vi "myRIO_BRig_Host_formatData_getHeaders_dataTrial.vi"() -> (3 "output_stringArray_dataTrial":string[](array[string]))   [LabVIEW 2014]
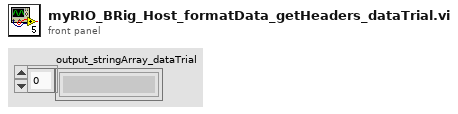
[diagram p1: front panel]
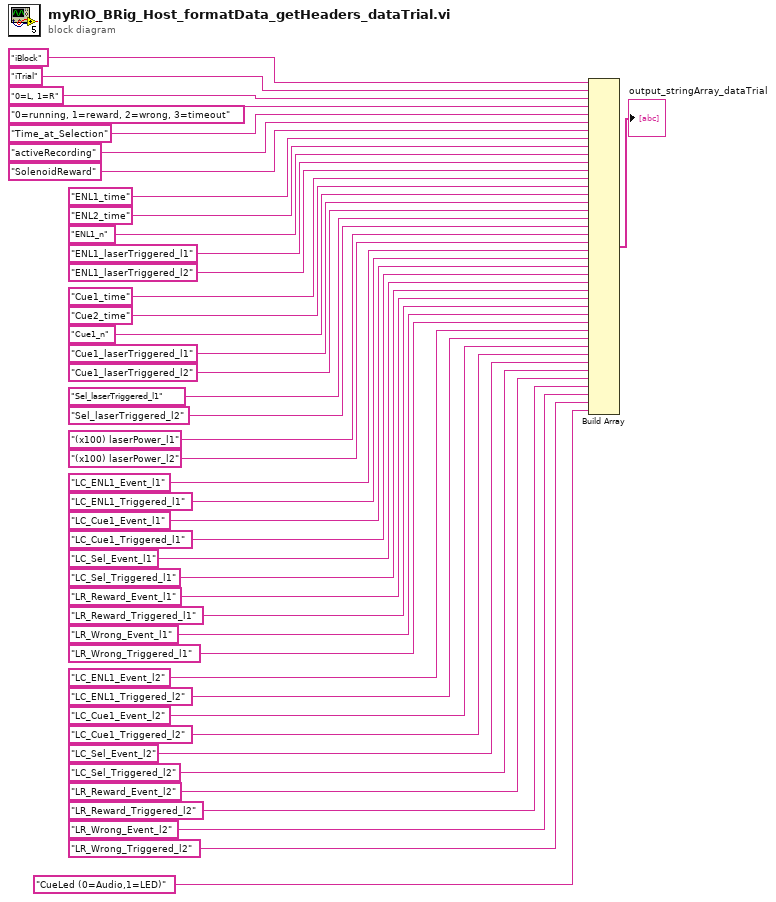
[diagram p0: block diagram]
diagram:
  n1 = Build Array("iBlock", "iTrial", "0=L, 1=R", "0=running, 1=reward, 2=wrong, 3=timeout", "Time_at_Selection", "activeRecording" ("element"), "SolenoidReward" ("element"), "ENL1_time", "ENL2_time", "ENL1_n", "ENL1_laserTriggered_l1", "ENL1_laserTriggered_l2", "Cue1_time", "Cue2_time", "Cue1_n", "Cue1_laserTriggered_l1", "Cue1_laserTriggered_l2", "Sel_laserTriggered_l1", "Sel_laserTriggered_l2", "(x100) laserPower_l1" ("element"), "(x100) laserPower_l2" ("element"), "LC_ENL1_Event_l1", "LC_ENL1_Triggered_l1", "LC_Cue1_Event_l1", "LC_Cue1_Triggered_l1", "LC_Sel_Event_l1", "LC_Sel_Triggered_l1", "LR_Reward_Event_l1", "LR_Reward_Triggered_l1", "LR_Wrong_Event_l1", "LR_Wrong_Triggered_l1", "LC_ENL1_Event_l2", "LC_ENL1_Triggered_l2", "LC_Cue1_Event_l2", "LC_Cue1_Triggered_l2", "LC_Sel_Event_l2", "LC_Sel_Triggered_l2", "LR_Reward_Event_l2", "LR_Reward_Triggered_l2", "LR_Wrong_Event_l2", "LR_Wrong_Triggered_l2", "CueLed (0=Audio,1=LED)") -> (→"output_stringArray_dataTrial":string[])
